vi "RichToFlatcif_channelcore_DestroyFIFOInstanceRequest.vi"(5 "OutputClusterType":T1, 11 "InputCluster":T2) -> (3 "OutputCluster":T1)   [LabVIEW 2021, in "CIFCoreChannel_server.lvlib"]
uses:
  CIFCoreChannel_server.lvlib
  cif_channelcore_DestroyFIFOInstanceRequest.ctl
  cif_channelcore_DestroyFIFOInstanceRequest_Flat.ctl
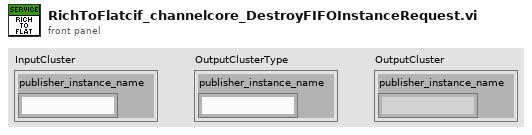
[diagram p1: front panel]
types:
  T1 = typedef "CIFCoreChannel_server.lvlib/cif_channelcore_DestroyFIFOInstanceRequest_Flat.ctl" = cluster{"publisher_instance_name":string}
  T2 = typedef "CIFCoreChannel_server.lvlib/cif_channelcore_DestroyFIFOInstanceRequest.ctl" = cluster{"publisher_instance_name":string}
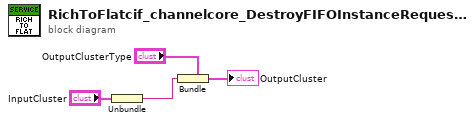
[diagram p0: block diagram]
diagram:
  n1 = Unbundle "Unbundle"("InputCluster") -> ("publisher_instance_name"=w1:string)
  n2 = Bundle "Bundle"(cluster="OutputClusterType", "publisher_instance_name"=w1) -> (→"OutputCluster":T1)
